vi "8742Control.vi"   [LabVIEW 2022 SP3]
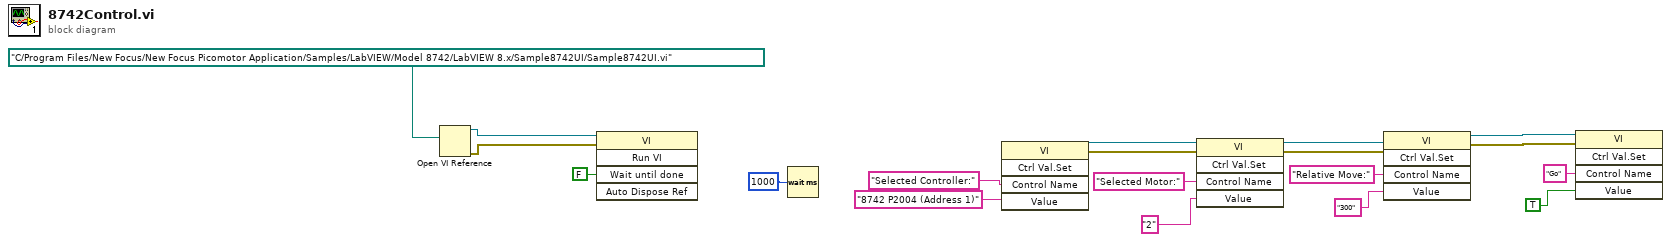
[diagram p0: block diagram]
diagram:
  n1 = Open VI Reference(vi path=path "C:/Program Files/New Focus/New Focus Picomotor Application/Samples/LabVIEW/Model 8742/LabVIEW 8.x/Sample8742UI/Sample8742UI.vi") -> (vi reference=w11:refnum<vi>, error out=w10:errorcluster)  [unwired: 5 in]
  n2 = invoke class="VI" method="Run VI"(reference=w11, error in=w10, "Wait until done"=FALSE ("Wait Until Done")) -> ()  [unwired: 2 in, 5 out]
  n3 = Wait (ms)(milliseconds to wait=u32 1000) -> ()  [unwired: 1 out]
  n4 = invoke class="VI" method="Ctrl Val.Set"("Control Name"="Selected Controller:", "Value"="8742 P2004 (Address 1)") -> (reference out=w16:refnum<vi>, error out=w15:errorcluster)  [unwired: 3 in, 3 out]
  n5 = invoke class="VI" method="Ctrl Val.Set"(reference=w16, error in=w15, "Control Name"="Selected Motor:", "Value"="2" ("Control Name")) -> (reference out=w13:refnum<vi>, error out=w12:errorcluster)  [unwired: 1 in, 3 out]
  n6 = invoke class="VI" method="Ctrl Val.Set"(reference=w13, error in=w12, "Control Name"="Relative Move:", "Value"="300" ("Control Name")) -> (reference out=w6:refnum<vi>, error out=w7:errorcluster)  [unwired: 1 in, 3 out]
  n7 = invoke class="VI" method="Ctrl Val.Set"(reference=w6, error in=w7, "Control Name"="Go", "Value"=TRUE) -> ()  [unwired: 1 in, 5 out]
